vi "M-686 Start Up.vi"(0 "VISA Ref":refnum<visa-resource-name>, 7 "Axes Names":string[](array[string]), 11 "Error In":errorcluster) -> (4 "VISA Ref Dup":refnum<visa-resource-name>, 15 "Error Out":errorcluster)   [LabVIEW 2020]
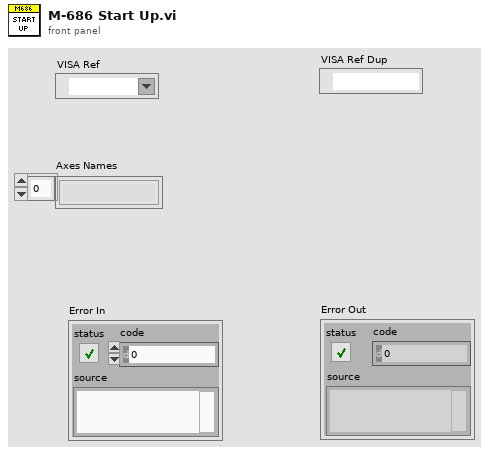
[diagram p1: front panel]
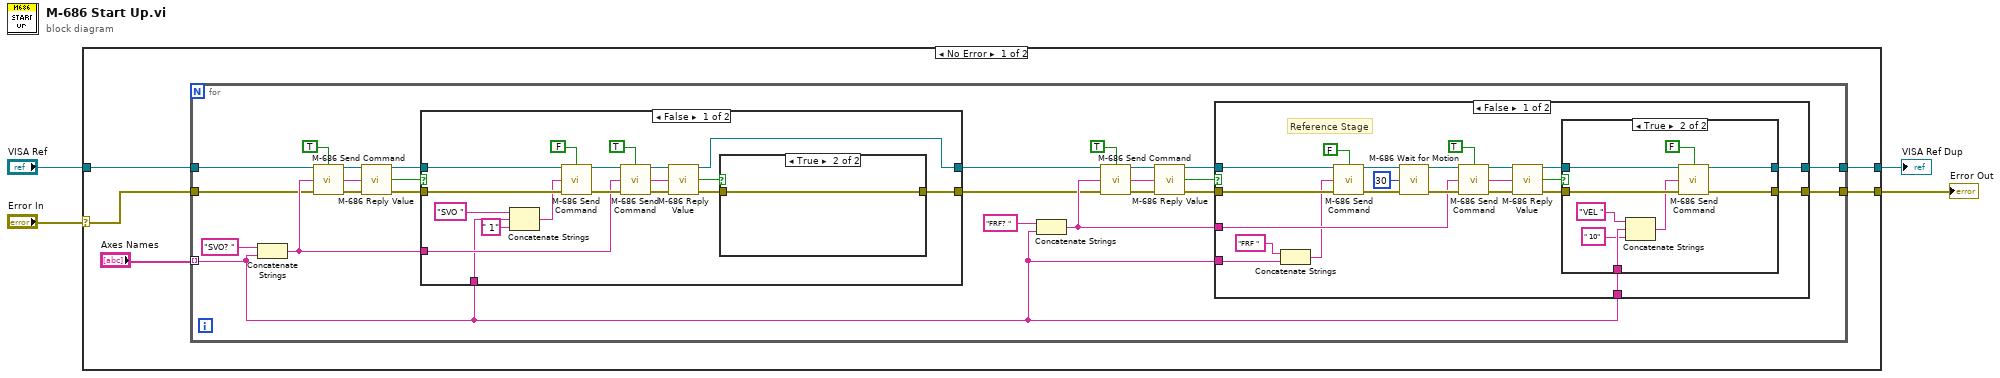
[diagram p0: block diagram]
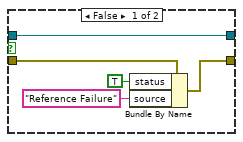
[diagram p2: hidden frame]
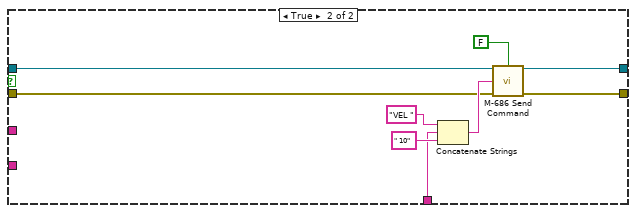
[diagram p3: hidden frame]
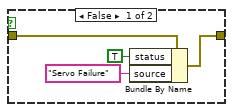
[diagram p4: hidden frame]
diagram:
  n1 = case shown="No Error" "Error In" {
    selector: "Error In" -> [w8 w105]
    tunnel: "VISA Ref" -> [w9 w106]
    tunnel: [w7 w106] -> w2
    tunnel: [w6 w105] -> w1
    frame No Error {
      n2 = for {
        tunnel: w8 -> [w24]
        tunnel: [w12] -> w6
        tunnel: w9 -> [w25]
        tunnel: [w13] -> w7
        tunnel: "Axes Names" -> [w10] mode=indexing
        n3 = Concatenate Strings("SVO? " ("Command"), w10) -> (w26:string)
        n4 = call "M-686 Send Command.vi"("VISA Ref"=w25, "Wait for Reply (T)"=TRUE, "Command"=w26, "Error In"=w24) -> ("VISA Ref Dup"=w33:refnum<visa-resource-name>, "Reply"=w32:string, "Error Out"=w31:errorcluster)  [unwired: 8 in, 1 out]
        n5 = call "M-686 Reply Value.vi"("VISA Pass Thru"=w33, "Cmd Reply"=w32, "Error In"=w31) -> ("VISA Ref Dup"=w29:refnum<visa-resource-name>, "Bool"=w30:bool, "Error Out"=w28:errorcluster)  [unwired: 9 in, 1 out]
        n6 = case shown="False" w30 {
          tunnel: w29 -> [w96 w104]
          tunnel: w28 -> [w95 w103]
          tunnel: [w86 w103] -> w11
          tunnel: [w85 w104] -> w14
          tunnel: w26 -> [w84 _]
          tunnel: w10 -> [w82 _]
          frame False {
            n7 = Concatenate Strings("SVO " ("string"), w82, " 1" ("string")) -> (w80:string)
            n8 = call "M-686 Send Command.vi"("VISA Ref"=w96, "Wait for Reply (T)"=FALSE, "Command"=w80, "Error In"=w95) -> ("VISA Ref Dup"=w90:refnum<visa-resource-name>, "Error Out"=w89:errorcluster)  [unwired: 8 in, 2 out]
            n9 = call "M-686 Send Command.vi"("VISA Ref"=w90, "Wait for Reply (T)"=TRUE, "Command"=w84, "Error In"=w89) -> ("VISA Ref Dup"=w92:refnum<visa-resource-name>, "Reply"=w93:string, "Error Out"=w94:errorcluster)  [unwired: 8 in, 1 out]
            n10 = call "M-686 Reply Value.vi"("VISA Pass Thru"=w92, "Cmd Reply"=w93, "Error In"=w94) -> ("VISA Ref Dup"=w85:refnum<visa-resource-name>, "Bool"=w88:bool, "Error Out"=w87:errorcluster)  [unwired: 9 in, 1 out]
            n11 = case shown="True" w88 {
              tunnel: w87 -> [w101 w102]
              tunnel: [w98 w102] -> w86
              frame False {
                n12 = Bundle By Name(cluster=w101, "status"=TRUE, "source"="Servo Failure") -> (w98:errorcluster)
              }
              frame True {
              }
            }
          }
          frame True {
          }
        }
        n13 = Concatenate Strings("FRF? " ("Command"), w10) -> (w17:string)
        n14 = call "M-686 Send Command.vi"("VISA Ref"=w14, "Wait for Reply (T)"=TRUE, "Command"=w17, "Error In"=w11) -> ("VISA Ref Dup"=w21:refnum<visa-resource-name>, "Reply"=w23:string, "Error Out"=w22:errorcluster)  [unwired: 8 in, 1 out]
        n15 = call "M-686 Reply Value.vi"("VISA Pass Thru"=w21, "Cmd Reply"=w23, "Error In"=w22) -> ("VISA Ref Dup"=w18:refnum<visa-resource-name>, "Bool"=w20:bool, "Error Out"=w19:errorcluster)  [unwired: 9 in, 1 out]
        n16 = case shown="False" w20 {
          tunnel: w19 -> [w55 w74]
          tunnel: w18 -> [w56 w75]
          tunnel: [w36 w72] -> w13
          tunnel: [w42 w71] -> w12
          tunnel: w17 -> [w41 _]
          tunnel: w10 -> [w40 _]
          tunnel: w10 -> [w35 w73]
          frame False {
            # "Reference Stage"
            n17 = Concatenate Strings("FRF " ("Command"), w40) -> (w38:string)
            n18 = call "M-686 Send Command.vi"("VISA Ref"=w56, "Wait for Reply (T)"=FALSE, "Command"=w38, "Error In"=w55) -> ("VISA Ref Dup"=w52:refnum<visa-resource-name>, "Error Out"=w53:errorcluster)  [unwired: 8 in, 2 out]
            n19 = call "M-686 Wait for Motion.vi"("VISA Ref"=w52, "Timeout (s)"=30, "Error In"=w53) -> ("VISA Ref Dup"=w46:refnum<visa-resource-name>, "Error Out"=w45:errorcluster)  [unwired: 11 in]
            n20 = call "M-686 Send Command.vi"("VISA Ref"=w46, "Wait for Reply (T)"=TRUE, "Command"=w41, "Error In"=w45) -> ("VISA Ref Dup"=w50:refnum<visa-resource-name>, "Reply"=w48:string, "Error Out"=w49:errorcluster)  [unwired: 8 in, 1 out]
            n21 = call "M-686 Reply Value.vi"("VISA Pass Thru"=w50, "Cmd Reply"=w48, "Error In"=w49) -> ("VISA Ref Dup"=w37:refnum<visa-resource-name>, "Bool"=w44:bool, "Error Out"=w43:errorcluster)  [unwired: 9 in, 1 out]
            n22 = case shown="True" w44 {
              tunnel: w43 -> [w61 w67]
              tunnel: [w58 w66] -> w42
              tunnel: w37 -> [w57 w69]
              tunnel: [w57 w68] -> w36
              tunnel: w35 -> [_ w64]
              frame False {
                n23 = Bundle By Name(cluster=w61, "status"=TRUE, "source"="Reference Failure") -> (w58:errorcluster)
              }
              frame True {
                n24 = Concatenate Strings("VEL " ("Command"), w64, " 10" ("string")) -> (w62:string)
                n25 = call "M-686 Send Command.vi"("VISA Ref"=w69, "Wait for Reply (T)"=FALSE, "Command"=w62, "Error In"=w67) -> ("VISA Ref Dup"=w68:refnum<visa-resource-name>, "Error Out"=w66:errorcluster)  [unwired: 8 in, 2 out]
              }
            }
          }
          frame True {
            n26 = Concatenate Strings("VEL " ("Command"), w73, " 10" ("string")) -> (w79:string)
            n27 = call "M-686 Send Command.vi"("VISA Ref"=w75, "Wait for Reply (T)"=FALSE, "Command"=w79, "Error In"=w74) -> ("VISA Ref Dup"=w72:refnum<visa-resource-name>, "Error Out"=w71:errorcluster)  [unwired: 8 in, 2 out]
          }
        }
      }
    }
    frame Error {
    }
  }
  "Error Out" <- w1
  "VISA Ref Dup" <- w2
